vi "configure.vi"(8 "error in (no error)":errorcluster, 11 "ExperimentControllerDL090130Interval in":refnum<class "ExperimentControllerDL090130Interval.lvclass">) -> (0 "error out":errorcluster, 3 "ExperimentControllerDL090130Interval out":refnum<class "ExperimentControllerDL090130Interval.lvclass">)   [LabVIEW 2010, in "ExperimentControllerDL090130Interval.lvclass"]
doc: "The dynamic dispatch version of this VI loads and displays the configuration file associated with the plug-in object. The user modify and save the configuration data."
uses:
  ExperimentControllerDL090130Interval.lvclass
  common/xcontrols/XComponentSpecification/XComponentSpecification/XComponentSpecification.xctl
  ExperimentControllerDL090130Interval.lvclass/ExperimentControllerDL090130Interval.ctl
  common/classes/ErrorController/ErrorController/class_data.vi
  common/classes/GenericComponent/GenericComponent/GenericComponent.lvclass
  common/classes/ErrorController/ErrorController/ErrorController.lvclass
panel:
  in  "cancel button":bool
  in  "save button":bool
  out "Configuration":string
  in  "Tab Control":enum32{"Description", "Sweep"}(tab)
  in  "sweep spec":T1(xcontrol)
  # "Configure ExperimentControllerDL090130Interval"
  # "This experimentController executes an image acquisition N times at a specified interval."
  # "If you don't specify a Sweep below, the image acquisition at each is performed by the already active imagingMode and its respective configuration and settings. \n\nIn contrast, if you specify a Sweep below, the configuration of the Sweep determines the image acqusition at each period. The sweep can consist of whole sequence of imagingModes, each with its own configuration and settings - thereby allowing automation of image acquisition."
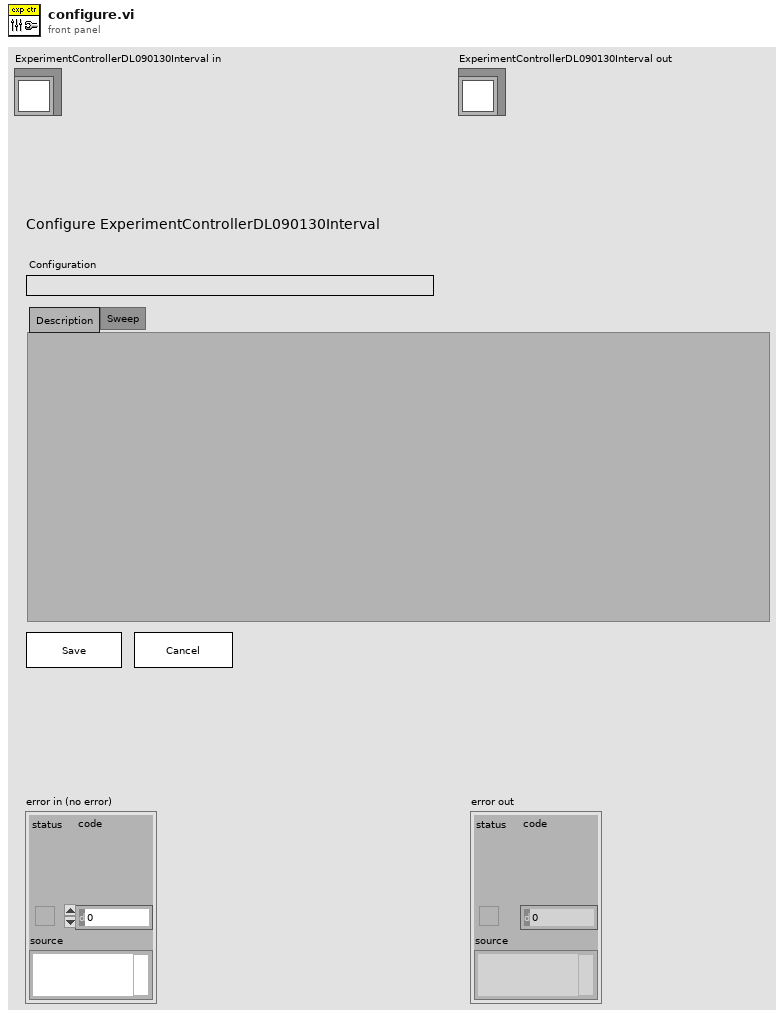
[diagram p1: front panel]
types:
  T1 = cluster{"class path":string, "configuration":string, "label":string, "settings name":string}
  T2 = typedef "plugin_specification.ctl" = cluster{"class path":string, "configuration":string, "label":string, "settings name":string}
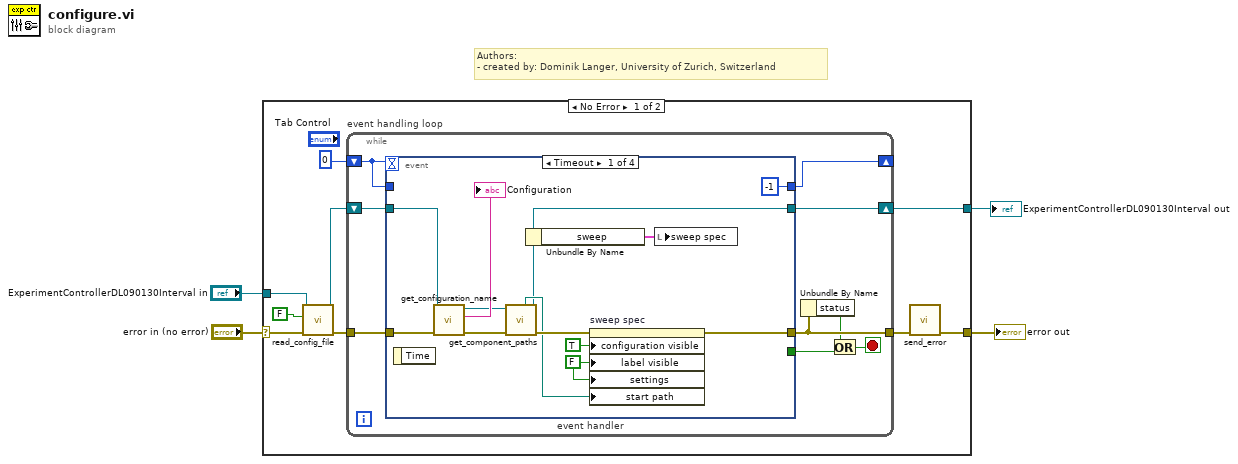
[diagram p0: block diagram]
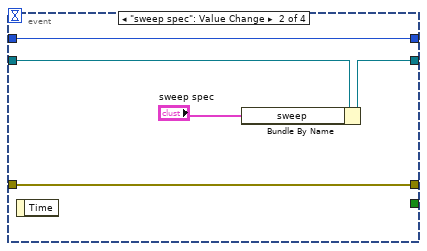
[diagram p2: hidden frame]
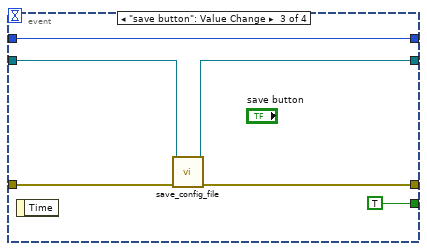
[diagram p3: hidden frame]
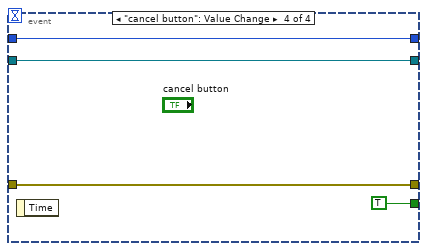
[diagram p4: hidden frame]
diagram:
  # "Authors: \n- created by: Dominik Langer, University of Zurich, Switzerland"
  n1 = case shown="No Error" "error in (no error)" {
    selector: "error in (no error)" -> [w12 w51]
    tunnel: "ExperimentControllerDL090130Interval in" -> [w10 w52]
    tunnel: [w6 w51] -> w2
    tunnel: [w8 w52] -> w1
    frame No Error {
      n2 = call-dynamic "read_config_file.vi"("error in (no error)"=w12, "force load?"=FALSE, "GenericPlugin in"=w10) -> ("error out"=w11:errorcluster, "GenericPlugin out"=w9:refnum<class "ExperimentControllerDL090130Interval.lvclass">)  [unwired: 7 in]
      n3 = while "event handling loop" {
        shift-right: [w20] -> w8
        shift-left: w9 -> [w21]
        shift-right: [w18] -> _
        shift-left: 0 -> [w19]
        tunnel: w11 -> [w22]
        tunnel: [w17] -> w5
        stop <- w16 stop-if-true
        n4 = event "event handler" shown="[0] Timeout" {
          selector: _ -> [_ _ _ _]
          dyn-events: _ -> [_ _ _ _]
          timeout: w19 -> [_ _ _ _]
          tunnel: w22 -> [w35 w40 w45 w49]
          tunnel: w21 -> [w34 w39 w41 w50]
          tunnel: [w23 w38 w43 w50] -> w20
          tunnel: [w30 w40 w44 w49] -> w17
          tunnel: [_ _ TRUE TRUE] -> w14
          tunnel: [-1 w37 w42 w47] -> w18
          tunnel: w19 -> [_ w37 w42 w47]
          event Timeout {
            w28 = FALSE ("label visible")
            n5 = event-data() -> ()  [unwired: 1 in, 1 out]
            n6 = call "get_configuration_name.vi"("error in (no error)"=w35, "GenericPlugin.lvclass in"=w34) -> ("error out"=w27:errorcluster, "configuration name"=→"Configuration":string, "GenericPlugin.lvclass out"=w24:refnum<class "ExperimentControllerDL090130Interval.lvclass">)  [unwired: 7 in]
            n7 = call-dynamic "get_component_paths.vi"("error in (no error)"=w27, "GenericComponent in"=w24) -> ("error out"=w26:errorcluster, "GenericComponent out"=w23:refnum<class "ExperimentControllerDL090130Interval.lvclass">, "component type directory"=w25:path)  [unwired: 4 in, 3 out]
            n8 = Unbundle By Name(w23) -> ("sweep"=w31:T2)
            n9 = property on="sweep spec" class="XComponentSpecification (strict"(error in=w26, "configuration visible"=TRUE, "label visible"=w28, "settings"=w28, "start path"=w25) -> (error out=w30:errorcluster)  [unwired: 1 in, 1 out]
            n10 = local write "sweep spec"(w31) -> ()
          }
          event "sweep spec": Value Change {
            n11 = event-data() -> ()  [unwired: 1 in, 1 out]
            n12 = Bundle By Name(cluster=w39, "sweep"="sweep spec") -> (w38:refnum<class "ExperimentControllerDL090130Interval.lvclass">)
          }
          event "save button": Value Change {
            n13 = event-data() -> ()  [unwired: 1 in, 1 out]
            n14 = call-dynamic "save_config_file.vi"("error in (no error)"=w45, "GenericPlugin in"=w41) -> ("error out"=w44:errorcluster, "GenericPlugin out"=w43:refnum<class "ExperimentControllerDL090130Interval.lvclass">)  [unwired: 8 in]
          }
          event "cancel button": Value Change {
            n15 = event-data() -> ()  [unwired: 1 in, 1 out]
          }
        }
        n16 = Unbundle By Name(w17) -> ("status"=w15:bool)
        n17 = Or(x=w15, y=w14) -> (x .or. y?=w16:bool)
      }
      n18 = call "send_error.vi"("error in (no error)"=w5) -> ("error out"=w6:errorcluster)  [unwired: 10 in]
    }
    frame Error {
    }
  }
  "error out" <- w2
  "ExperimentControllerDL090130Interval out" <- w1
